vi "I2C Read.vi"(6 "Timeout (1000 ms)":u16=1000, 8 "error in (no error)":errorcluster, 10 "# Bytes to Read":u8, 11 "LINX-PCA9865 PWM in":refnum<class "LINX-PCA9865 PWM.lvclass">) -> (0 "error out":errorcluster, 2 "Bytes Read":u8[](array[numeric]), 3 "LINX-PCA9865 PWM out":refnum<class "LINX-PCA9865 PWM.lvclass">)   [LabVIEW 2019, in "LINX-PCA9865 PWM.lvclass"]
uses:
  LINX-PCA9865 PWM.lvclass
  LINX-PCA9865 PWM.lvclass/LINX-PCA9865 PWM.ctl
  <vilib>/MakerHub/LINX/LMH-LINX.lvlib
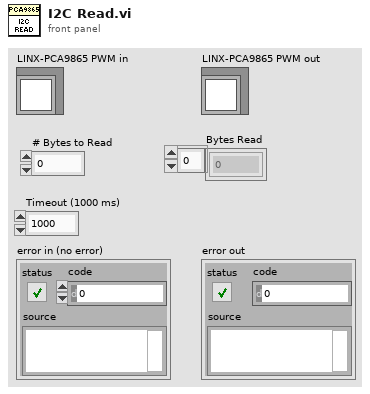
[diagram p1: front panel]
types:
  T1 = typedef "LMH-LINX.lvlib/LINX Ref.ctl" = cluster{"IO":T2, "Interface":T3, "LINX Device Config":T4}
  T2 = typedef "LMH-LINX.lvlib/Platform.ctl" = enum16{"Remote", "Local"}
  T3 = typedef "LMH-LINX.lvlib/Interface.ctl" = enum16{"Serial", "TCP"}
  T4 = typedef "LMH-LINX.lvlib/Device.lvlib/LINX Device Config.ctl" = cluster{"Interface":T3, "COM Port":refnum<visa-resource-name>, "TCP Configuration":T5, "Device Family":u8, "Device ID":u8, "Device Name":string, "TCP Ref":refnum<k5>, "Channels":T6}
  T5 = typedef "LMH-LINX.lvlib/Device.lvlib/TCP Config.ctl" = cluster{"IP Address":string, "Port":u16}
  T6 = typedef "LMH-LINX.lvlib/Channels.ctl" = cluster{"DI":u8[], "DO":u8[], "AI":u8[], "AO":u8[], "PWM":u8[], "QE":u8[], "UART":u8[], "I2C 2":u8[], "SPI":u8[], "CAN":u8[], "Servo":u8[], "AI Ref (V)":dbl, "AI Resolution (Bits)":u8, "AO Ref (V)":dbl, "AO Resolution (Bits)":u8}
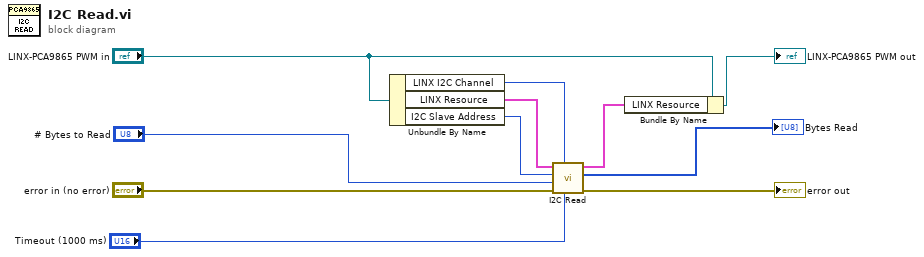
[diagram p0: block diagram]
diagram:
  n1 = Unbundle By Name("LINX-PCA9865 PWM in") -> ("LINX I2C Channel"=w9:u8, "LINX Resource"=w10:T1, "I2C Slave Address"=w11:u8)
  n2 = call <vilib>:"I2C Read.vi"("Timeout (1000 ms)"="Timeout (1000 ms)", "I2C Channel"=w9, "Error In"="error in (no error)", "Bytes To Read"="# Bytes to Read", "I2C Slave Address (0)"=w11, "LINX Resource"=w10) -> ("Error Out"=→"error out":errorcluster, "Data"=→"Bytes Read":u8[], "LINX Resource"=w7:T1)  [unwired: 3 in]
  n3 = Bundle By Name(cluster="LINX-PCA9865 PWM in", "LINX Resource"=w7) -> (→"LINX-PCA9865 PWM out":refnum<class "LINX-PCA9865 PWM.lvclass">)
